vi "Generate Reports Post-DAQ.vi"() -> ()   [LabVIEW 2015]
panel:
  out "Total Test Energies":dbl[](array[numeric])
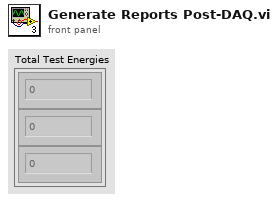
[diagram p1: front panel]
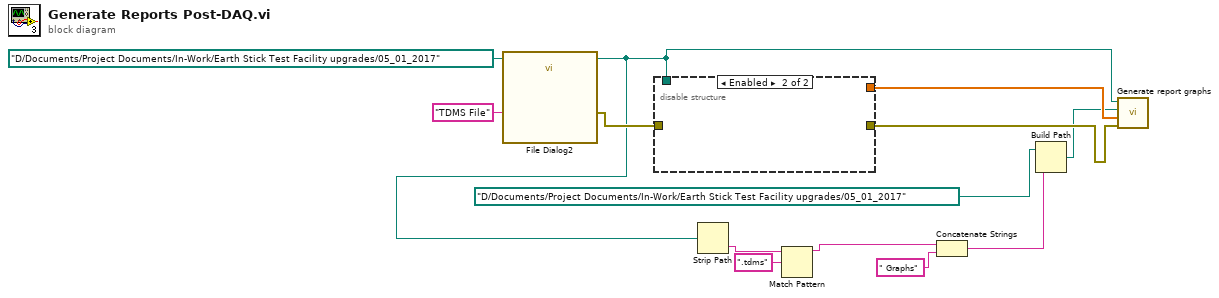
[diagram p0: block diagram]
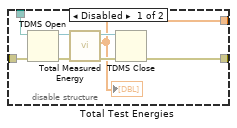
[diagram p2: hidden frame]
diagram:
  n1 = call "File Dialog2"("start path"=path "D:/Documents/Project Documents/In-Work/Earth Stick Test Facility upgrades/05_01_2017", "prompt"="TDMS File") -> ("selected path"=w9:path, "error out"=w11:errorcluster)  [unwired: 10 in, 2 out]
  n2 = disable-structure shown="Enabled" {
    disable-tunnel: [w17 _] -> w13
    disable-tunnel: w11 -> [w16 _]
    disable-tunnel: w9 -> [w15 _]
    disable-tunnel: [w14 _] -> w4
    frame Disabled {
      n3 = TDMS Open(8:w16, 11:w15) -> (0:w18:errorcluster, 3:w21:refnum<k34>)  [unwired: 5 in]
      n4 = call "Total Measured Energy.vi"("error in (no error)"=w18, "tdms file"=w21) -> ("error out"=w19:errorcluster, "Total Test Energies (J)"=w17:dbl[], "tdms file out"=w20:refnum<k34>)  [unwired: 5 in, 2 out]
      "Total Test Energies" <- w17
      n5 = TDMS Close(8:w19, 11:w20) -> (0:w14:errorcluster)  [unwired: 1 out]
    }
    frame Enabled {
    }
  }
  n6 = Strip Path(path=w9) -> (name=w7:string)  [unwired: 1 out]
  n7 = Match Pattern(string=w7, regular expression=".tdms") -> (before substring=w5:string)  [unwired: 1 in, 3 out]
  n8 = Concatenate Strings(w5, " Graphs" ("string")) -> (w2:string)
  n9 = Build Path(base path=path "D:/Documents/Project Documents/In-Work/Earth Stick Test Facility upgrades/05_01_2017" ("start path"), name or relative path=w2) -> (appended path=w1:path)
  n10 = call "Generate report graphs.vi"("error in (no error)"=w4, "Test Energies"=w13, "report file path"=w1, "file path"=w9) -> ()  [unwired: 7 in, 1 out]
